vi "Dispose.vi"(8 "error in (no error)":errorcluster, 11 "FaceRecognition in":refnum<class "FaceRecognition.lvclass">) -> (0 "error out":errorcluster, 3 "FaceRecognition out":refnum<class "FaceRecognition.lvclass">)   [LabVIEW 2020, in "FaceRecognitionDotNet.lvlib" / "FaceRecognition.lvclass"]
uses:
  FaceRecognition.lvclass
  FaceRecognition.lvclass/FaceRecognition.ctl
  dll/FaceRecognitionDotNet.dll
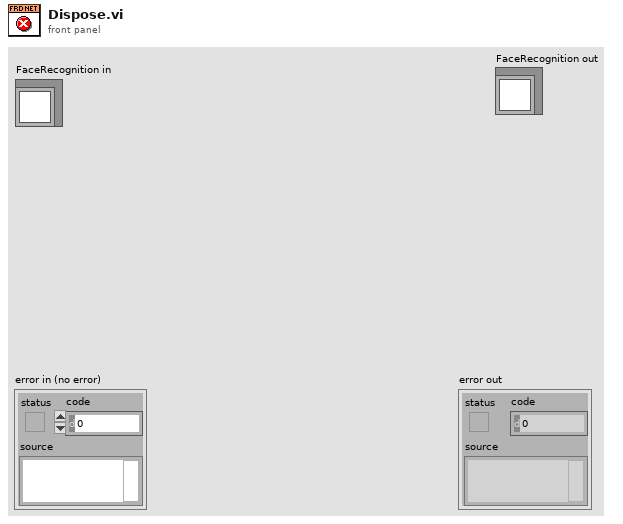
[diagram p1: front panel]
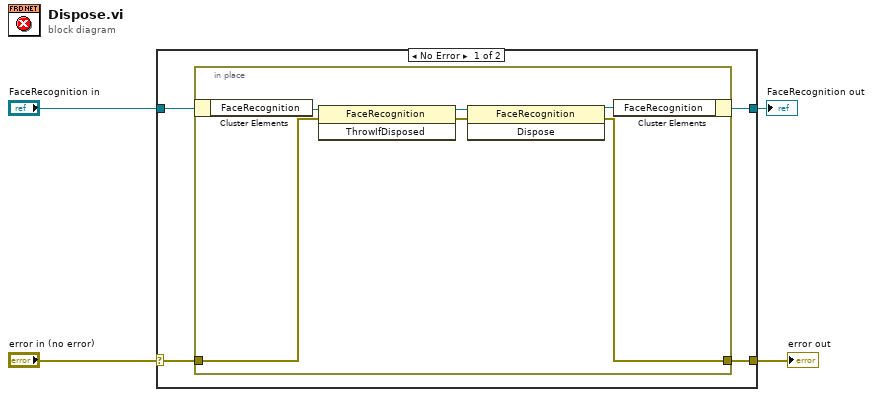
[diagram p0: block diagram]
diagram:
  n1 = case shown="No Error" "error in (no error)" {
    selector: "error in (no error)" -> [w6 w16]
    tunnel: [w5 w16] -> w3
    tunnel: [w7 w15] -> w1
    tunnel: "FaceRecognition in" -> [w8 w15]
    frame No Error {
      n2 = in-place {
        in-place-border: w6 -> [w13]
        in-place-border: [w10] -> w5
        n3 = in-place-cluster #1(w8) -> ("FaceRecognition"=w14:refnum<k24>)
        n4 = invoke class="FaceRecognition" method="ThrowIfDisposed"(reference=w14, error in=w13) -> (reference out=w12:refnum<k24>, error out=w11:errorcluster)  [unwired: 1 in, 1 out]
        n5 = invoke class="FaceRecognition" method="Dispose"(reference=w12, error in=w11) -> (reference out=w9:refnum<k24>, error out=w10:errorcluster)  [unwired: 1 in, 1 out]
        n6 = in-place-cluster #1("FaceRecognition"=w9) -> (w7:refnum<class "FaceRecognition.lvclass">)
      }
    }
    frame Error {
    }
  }
  "error out" <- w3
  "FaceRecognition out" <- w1
